vi "Stanford Research 830 Acquire Measurement - Multiple Points.vi"() -> ()   [LabVIEW 2012]
doc: "This example shows how to configure the instrument to read multiple points on the Channel 1 Display."
uses:
  <instrlib>/Stanford Research 830/Public/Data/Read (Multiple Points).vi
  <instrlib>/Stanford Research 830/Stanford Research 830.lvlib
panel:
  in  "Internal Reference Frequency (1000 Hz)":dbl=1000.0
  in  "Channel 1 Display (0: X)":u16(ring) items=["X", "R", "X Noise", "Aux In 1", "Aux In 2"]
  in  "Sine Output Amplitude (1 V)":dbl=1.0
  in  "Reference Source (1: Internal)":u16(ring)=1 items=["External", "Internal"]
  in  "Input Coupling (0: AC)":u16(ring) items=["AC", "DC"]
  in  "Input Connection (0: Single-Ended Voltage)":u16(ring) items=["Single-Ended Voltage", "Differential Voltage", "1 MOhm Current Gain", "100 MOhm Current Gain"]
  in  "Number of Points (100)":u32=100
  out "Measurements":sgl[](array[numeric])
  in  "Sample Rate (10: 64 Hz)":u16(ring)=10 items=["62.5 mHz", "125 mHz", "250 mHz", "500 mHz", "1 Hz", "2 Hz", "4 Hz", "8Hz", "16 Hz", "32 Hz", "64 Hz", "128 Hz", "256 Hz", "512 Hz", "Trigger "]
  in  "VISA resource name":refnum<visa-resource-name>
  # "(c) 2006 National Instruments.  ALL RIGHTS RESERVED."
  # "Input Signal"
  # "Reference"
  # "Acquisition"
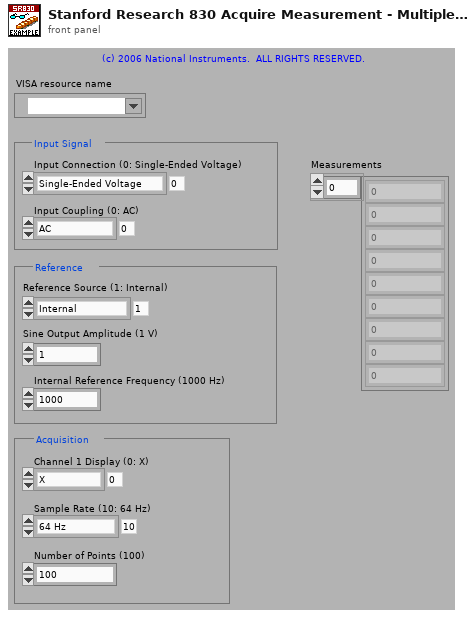
[diagram p1: front panel]
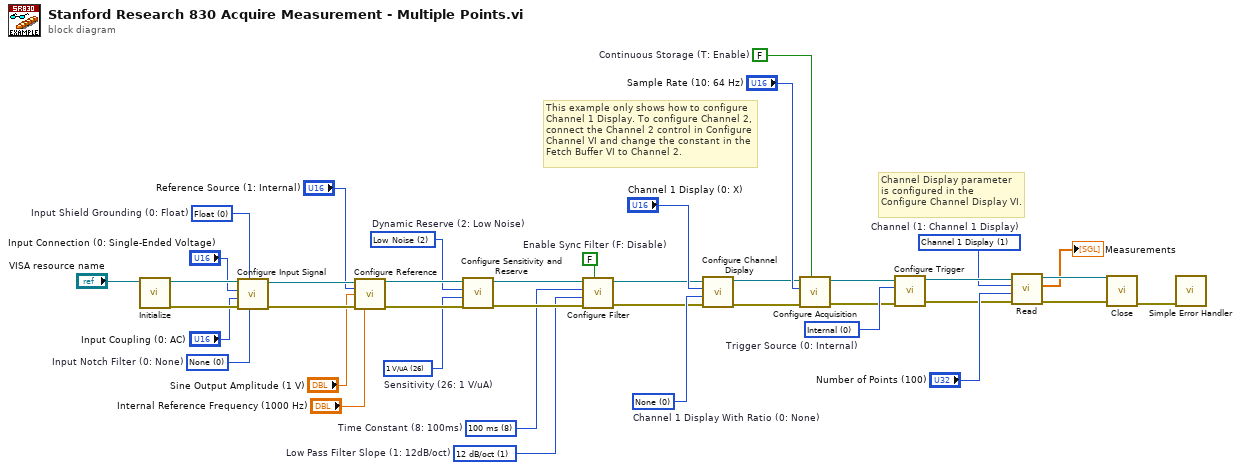
[diagram p0: block diagram]
diagram:
  w1 = FALSE  # Enable Sync Filter (F: Disable)
  w2 = u16 1 items=["6 dB/oct", "12 dB/oct", "18 db/oct", "24 dB/oct"]  # Low Pass Filter Slope (1: 12dB/oct)
  w3 = u16 8 items=["10 us", "30 us", "100 us", "300 us", "1 ms", "3 ms", "10 ms", "30 ms", "100 ms", "300 ms", "1 s", "3 s", "10 s", "30 s", "100 s", "300 s", "1 ks", "3 ks", "10 ks", "30 ks"]  # Time Constant (8: 100ms)
  w9 = u16 0 items=["None", "Aux In 1", "Aux In 2"]  # Channel 1 Display With Ratio (0: None)
  w13 = u16 1 items=["Channel 1 Display"=1, "Channel 2 Display"=2]  # Channel (1: Channel 1 Display)
  w15 = i16 26 items=["Auto Gain"=-1, "2 nV/fA"=0, "5 nV/fA"=1, "10 nV/fA"=2, "20 nV/fA"=3, "50 nV/fA"=4, "100 nV/fA"=5, "200 nV/fA"=6, "500 nV/fA"=7, "1 uV/pA"=8, "2 uV/pA"=9, "5 uV/pA"=10, "10 uV/pA"=11, "20 uV/pA"=12, "50 uV/pA"=13, "100 uV/pA"=14, "200 uV/pA"=15, "500 uV/pA"=16, "1 mV/nA"=17, "2 mV/nA"=18, "5 mV/nA"=19, "10 mV/nA"=20, "20 mV/nA"=21, "50 mV/nA"=22, "100 mV/nA"=23, "200 mV/nA"=24, "500 mV/mA"=25, "1 V/uA"=26]  # Sensitivity (26: 1 V/uA)
  w14 = i16 2 items=["Auto Reserve"=-1, "High Reserve"=0, "Normal"=1, "Low Noise"=2]  # Dynamic Reserve (2: Low Noise)
  w18 = u16 0 items=["None", "Line Notch", "2x Line Notch", "Both Notch Filters"]  # Input Notch Filter (0: None)
  w21 = u16 0 items=["Float", "Ground"]  # Input Shield Grounding (0: Float)
  w38 = u16 0 items=["Internal", "External"]  # Trigger Source (0: Internal)
  w36 = FALSE  # Continuous Storage (T: Enable)
  # "Channel Display parameter is configured in the Configure Channel Display VI."
  # "This example only shows how to configure Channel 1 Display. To configure Channel 2, connect the Channel 2 control in Configure Channel VI and change the constant in the Fetch Buffer VI to Channel 2."
  n1 = call <instrlib>:"Initialize.vi"("VISA resource name"="VISA resource name") -> ("error out"=w22:errorcluster, "VISA resource name out"=w23:refnum<visa-resource-name>)  [unwired: 9 in]
  n2 = call <instrlib>:"Configure Input Signal.vi"("Input Notch Filter (0: None)"=w18, "Input Shield Grounding (0: Float)"=w21, "error in (no error)"=w22, "Input Coupling (0: AC)"="Input Coupling (0: AC)", "Input Connection (0: Single-Ended Voltage)"="Input Connection (0: Single-Ended Voltage)", "VISA resource name"=w23) -> ("error out"=w26:errorcluster, "VISA resource name out"=w27:refnum<visa-resource-name>)  [unwired: 4 in]
  n3 = call <instrlib>:"Configure Reference.vi"("VISA resource name"=w27, "Reference Source (1: Internal)"="Reference Source (1: Internal)", "Sine Output Amplitude (1 V)"="Sine Output Amplitude (1 V)", "error in (no error)"=w26, "Internal Reference Frequency (1000 Hz)"="Internal Reference Frequency (1000 Hz)") -> ("VISA resource name out"=w24:refnum<visa-resource-name>, "error out"=w25:errorcluster)  [unwired: 9 in]
  n4 = call <instrlib>:"Configure Sensitivity and Reserve.vi"("error in (no error)"=w25, "Sensitivity (-1: Auto gain)"=w15, "Dynamic Reserve (-1: Auto Reserve)"=w14, "VISA resource name"=w24) -> ("error out"=w6:errorcluster, "VISA resource name out"=w7:refnum<visa-resource-name>)  [unwired: 6 in]
  n5 = call <instrlib>:"Configure Filter.vi"("Enable Sync Filter (F: Disable)"=w1, "error in (no error)"=w6, "Low Pass Filter Slope (1: 12dB/oct)"=w2, "Time Constant (8: 100ms)"=w3, "VISA resource name"=w7) -> ("error out"=w4:errorcluster, "VISA resource name out"=w5:refnum<visa-resource-name>)  [unwired: 5 in]
  n6 = call <instrlib>:"Configure Channel Display.vi"("error in (no error)"=w4, "Channel 1 Display With Ratio (0: None)"=w9, "Channel 1 Display (0: X)"="Channel 1 Display (0: X)", "VISA resource name"=w5) -> ("error out"=w11:errorcluster, "VISA resource name out"=w12:refnum<visa-resource-name>)  [unwired: 6 in]
  n7 = call <instrlib>:"Configure Acquisition.vi"("Continuous Storage (T: Enable)"=w36, "error in (no error)"=w11, "Sample Rate (0: 62.5 mHz)"="Sample Rate (10: 64 Hz)", "VISA resource name"=w12) -> ("error out"=w34:errorcluster, "VISA resource name out"=w35:refnum<visa-resource-name>)  [unwired: 6 in]
  n8 = call <instrlib>:"Configure Trigger.vi"("error in (no error)"=w34, "Trigger Source (0: Internal)"=w38, "VISA resource name"=w35) -> ("error out"=w31:errorcluster, "VISA resource name out"=w32:refnum<visa-resource-name>)  [unwired: 7 in]
  n9 = call-poly <instrlib>:"Read.vi"("error in (no error)"=w31, "Number of Points (100)"="Number of Points (100)", "Channel (1: Channel 1 Display)"=w13, "VISA resource name"=w32) -> ("error out"=w29:errorcluster, "Measurements"=→"Measurements":sgl[], "VISA resource name out"=w30:refnum<visa-resource-name>)  [unwired: 5 in]
  n10 = call <instrlib>:"Close.vi"("error in (no error)"=w29, "VISA resource name"=w30) -> ("error out"=w40:errorcluster)  [unwired: 9 in]
  n11 = call <vilib>:"Simple Error Handler.vi"("error in (no error)"=w40) -> ()  [unwired: 4 in, 5 out]
